vi "CmdGetStatsMeanValue.vi"(0 "PM Cmds In":refnum<k24>, 5 "Device Key In":string, 11 "error in":errorcluster) -> (4 "PM Cmds Out":refnum<k24>, 6 "Device Key Out":string, 8 "I/O Status":i32, 10 "Mean Value":sgl format="%^#_6g", 15 "error out":errorcluster)   [LabVIEW 2021]
uses:
  C:/_git/mantoles-dev-box/LabVIEW/sample-code/LabVIEW 2010/PowerMeterCommands.dll
  PowerMeterCommands.dll
panel:
  in  "mean":sgl
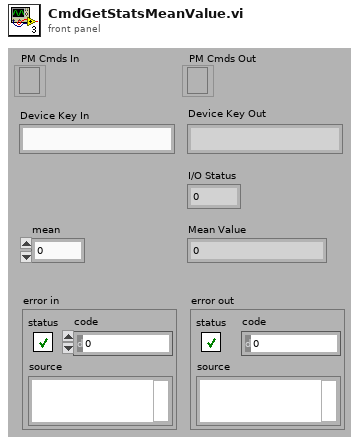
[diagram p1: front panel]
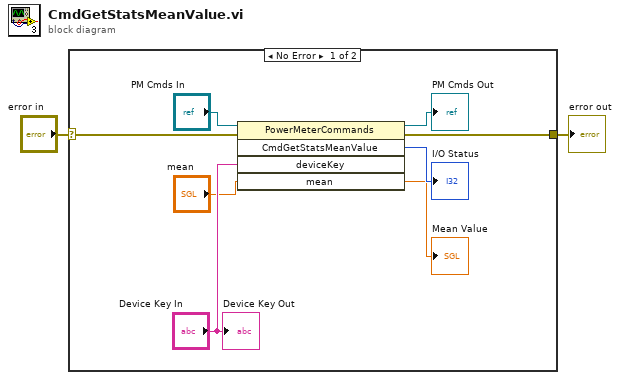
[diagram p0: block diagram]
diagram:
  n1 = case shown="No Error" "error in" {
    selector: "error in" -> [w7 w11]
    tunnel: [w9 w11] -> w2
    frame No Error {
      n2 = invoke class="PowerMeterCommands" method="CmdGetStatsMeanValue"(reference="PM Cmds In", error in=w7, "deviceKey"="Device Key In", "mean"="mean") -> (reference out=→"PM Cmds Out":refnum<k24>, error out=w9:errorcluster, "CmdGetStatsMeanValue"=→"I/O Status":i32, "mean"=→"Mean Value":sgl)  [unwired: 1 in, 1 out]
      "Device Key Out" <- "Device Key In"
    }
    frame Error {
    }
  }
  "error out" <- w2
